vi "stoperaseCI2_img.vi"   [LabVIEW 2013]
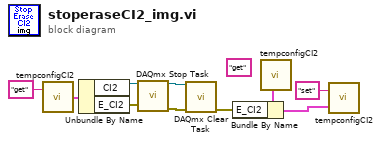
[diagram p0: block diagram]
diagram:
  (unwired) "get" ("command")
  n1 = call "tempconfigCI2.vi"("command"="get") -> ("Temp Config out"=w7:cluster{"CI2":refnum<k21>, "E_CI2":errorcluster})  [unwired: 1 in]
  n2 = Unbundle By Name(w7) -> ("CI2"=w6:refnum<k21>, "E_CI2"=w5:errorcluster)
  n3 = call <vilib>:"DAQmx Stop Task.vi"("task/channels in"=w6, "error in"=w5) -> ("task out"=w9:refnum<k21>, "error out"=w10:errorcluster)  [unwired: 12 in]
  n4 = call <vilib>:"DAQmx Clear Task.vi"("task in"=w9, "error in"=w10) -> ("error out"=w2:errorcluster)  [unwired: 13 in]
  n5 = call "tempconfigCI2.vi"() -> ("Temp Config out"=w3:cluster{"CI2":refnum<k21>, "E_CI2":errorcluster})  [unwired: 2 in]
  n6 = Bundle By Name(cluster=w3, "E_CI2"=w2) -> (w1:cluster{"CI2":refnum<k21>, "E_CI2":errorcluster})
  n7 = call "tempconfigCI2.vi"("Temp Config in"=w1, "command"="set") -> ()  [unwired: 1 out]
